vi "CPP-ZeroMonitor.vi"(4 "Scan Period":dbl format="%.2f", 5 "Previous Scan Value":dbl format="%.2f", 6 "Present scan array":dbl[](array[numeric]) format="%.2f", 7 "Value to Output":dbl format="%.2f", 8 "Ch Description":T1={"Ch Name"="Tunnel3:Pressures:", "Type"="", "Function"=enum."Analogue Input", "Ch State"=enum."On", "Calibration type"=enum."Raw", "A"=30.0, "B"=10.0, "C"=0.0, "D"=0.0, "Comments"="", "Address"={"Main"=0, "Ch."=0, "Sub"=0, "Port Name"=""}, "String"="", "Duty"=65535} {"Duty" format="%.0b"; "D" format="%#_5g"; "C" format="%#_5g"; "B" format="%#_5g"; "A" format="%#_5g"}, 9 "Ch names":string[](array[string])) -> (0 "Scan comment":string, 1 "Output":dbl=0.0037402657506766107)   [LabVIEW 2014]
doc: "Wrapper for CPP-ZerosMaintenance.vi\nChannels Names should have the format \"Tunnel#:Pressures:\" (e.g. Tunnel1:Pressures: or Tunnel3:Pressures:). A = SecondsToMonitor (intervall to determine if tunnel has been off long enough and to inspect zero drift. B = SecondsToAverage (averaging interval for transducer zeros)."
uses:
  ADAM Client/Sub VIs/ADAM Controls/Ch_description_ADAM.ctl
  ADAM Client/Sub VIs/ADAM Controls/Module_type_ADAM.ctl
  ADAM Client/Sub VIs/ADAM Controls/Function_ADAM.ctl
  ADAM Client/Sub VIs/ADAM Controls/Channel_State.ctl
  ADAM Client/Sub VIs/ADAM Controls/Calib_type_ADAM.ctl
  ADAM Client/Sub VIs/ADAM Controls/Address.ctl
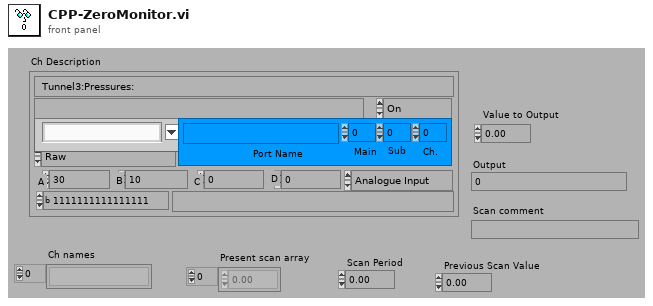
[diagram p1: front panel]
types:
  T1 = typedef "Ch_description_ADAM.ctl" = cluster{"Ch Name":string, "Type":T2, "Function":T3, "Ch State":T4, "Calibration type":T5, "A":dbl, "B":dbl, "C":dbl, "D":dbl, "Comments":string, "Address":T6, "String":string, "Duty":u16}
  T2 = typedef "Module_type_ADAM.ctl" = string
  T3 = typedef "Function_ADAM.ctl" = enum16{"Analogue Input", "Digital Input", "Event counter", "Event rate", "Analogue Output", "Digital Output", "Relay Output"}
  T4 = typedef "Channel_State.ctl" = enum16{"On", "Off", "Always On", "Always Off"}
  T5 = typedef "Calib_type_ADAM.ctl" = enum16{"Raw", "Bx + A", "Cx^2 + Bx + A", "Dx^3 + Cx^2 + Bx + A", "In Band", "Hi-Tec Q", "Hi-Tec M_dot", "Text"}
  T6 = typedef "Address.ctl" = cluster{"Main":i32, "Ch.":i32, "Sub":i32, "Port Name":string}
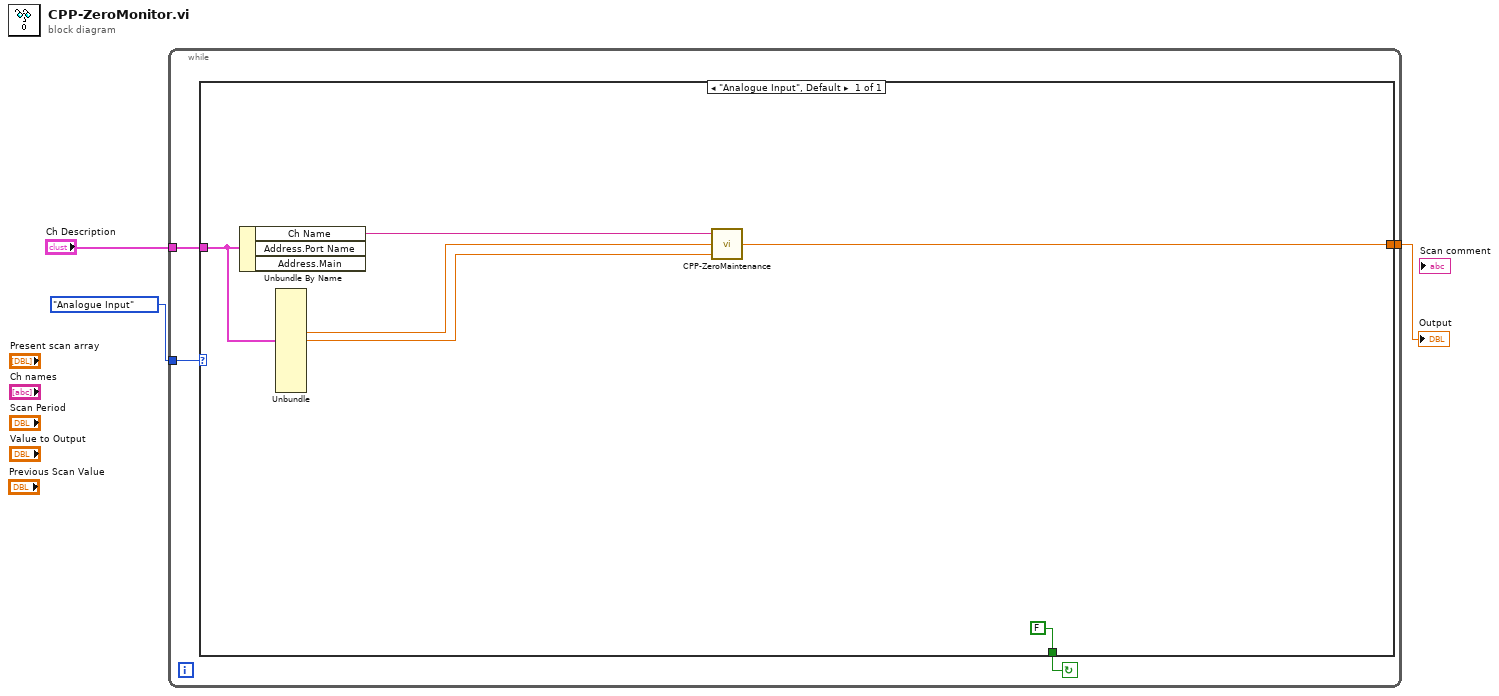
[diagram p0: block diagram]
diagram:
  n1 = while {
    tunnel: "Ch Description" -> [w7]
    tunnel: Function_ADAM."Analogue Input" ("Function") -> [w6]
    tunnel: [w4] -> w1
    stop <- w5 continue-if-true
    n2 = case shown="\"Analogue Input\", Default" w6 {
      tunnel: w7 -> [w13]
      tunnel: [FALSE] -> w5
      tunnel: [w8] -> w4
      frame "Analogue Input", Default {
        n3 = Unbundle By Name(w13) -> ("Ch Name"=w11:string)  [unwired: 2 out]
        n4 = Unbundle(w13) -> ("A"=w10:dbl, "B"=w9:dbl)  [unwired: 11 out]
        n5 = call "CPP-ZeroMaintenance.vi"("SecondsToAverage"=w9, "SecondsToMonitor"=w10, "Tunnel#:Pressures:"=w11) -> ("Time Elapsed (sec)"=w8:dbl)
      }
    }
  }
  "Output" <- w1
